vi "4.4 CSM API String to Numeric - TimeStamp.vi"() -> ()   [LabVIEW 2017]
uses:
  80786043-8302-4494-baed-a946b518dc40.vi
  b96edd05-43f6-4913-a4f3-d608f403e629.vi
  87278fde-cd95-4c12-a361-3a4a12f7c62e.vi
  36ad7d10-f589-4ebf-988f-4972958953c5.vi
  e1f6a09e-d061-4c8c-81e9-a26d802c807e.vi
  7cb491dc-0bc3-43bf-bfd1-0206b192279c.vi
  API-String-Arugments-Support/_Support/Convert API String Arguments to Data(variant).vi
  API-String-Arugments-Support/_Support/Data To API String Arguments.vi
  API-String-Arugments-Support/API String Arguments Support.lvlib
panel:
  out "output 4":T1={"Original"=timestamp(3779880873.3011937 s since 1904-01-01), "format string"="%<%Y-%m-%d %H:%M:%S>T", "CSM Timestamp Argument"="2023-10-11 22:54:33(%<%Y-%m-%d %H:%M:%S>T)", "Retrieved TimeStamp"=timestamp(3779880873 s since 1904-01-01), "Flatten String"="2023-10-11T14:54:33.000Z"}
  out "output 2":T2={"Argument String"="2023-10-31T14:49:39.597Z", "Type"=timestamp(0 s since 1904-01-01), "Retrieved TimeStamp"=timestamp(3781522179.597 s since 1904-01-01)}
  out "output 3":T3={"Original   "=timestamp(3781608579.597416 s since 1904-01-01), "Flatten String"="2023-10-31T14:49:39.597Z", "Type"=timestamp(0 s since 1904-01-01), "Retrieved TimeStamp"=timestamp(3781522179.597 s since 1904-01-01)}
  out "output 1":T2={"Argument String"="", "Type"=timestamp(0 s since 1904-01-01), "Retrieved TimeStamp"=timestamp(3839278850.481537 s since 1904-01-01)}
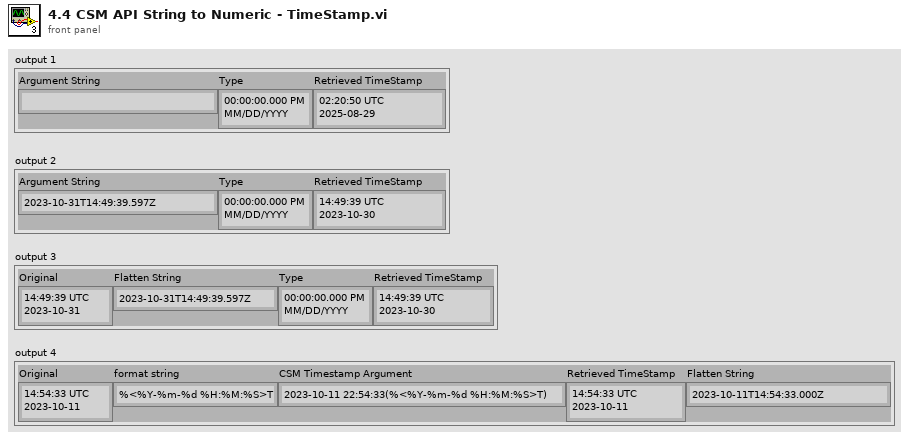
[diagram p1: front panel]
types:
  T1 = cluster{"Original":timestamp, "format string":string, "CSM Timestamp Argument":string, "Retrieved TimeStamp":timestamp, "Flatten String":string}
  T2 = cluster{"Argument String":string, "Type":timestamp, "Retrieved TimeStamp":timestamp}
  T3 = cluster{"Original   ":timestamp, "Flatten String":string, "Type":timestamp, "Retrieved TimeStamp":timestamp}
  T4 = cluster{"Empty String":string, "Type":timestamp, "Data":timestamp}
  T5 = cluster{"Arguments String":string, "Type":timestamp, "Data":timestamp}
  T6 = cluster{"Original   ":timestamp, "String":string, "Type":timestamp, "Data":timestamp}
  T7 = cluster{"Original":timestamp, "format string":string, "CSM Timestamp Argument":string, "Data":timestamp, "String":string}
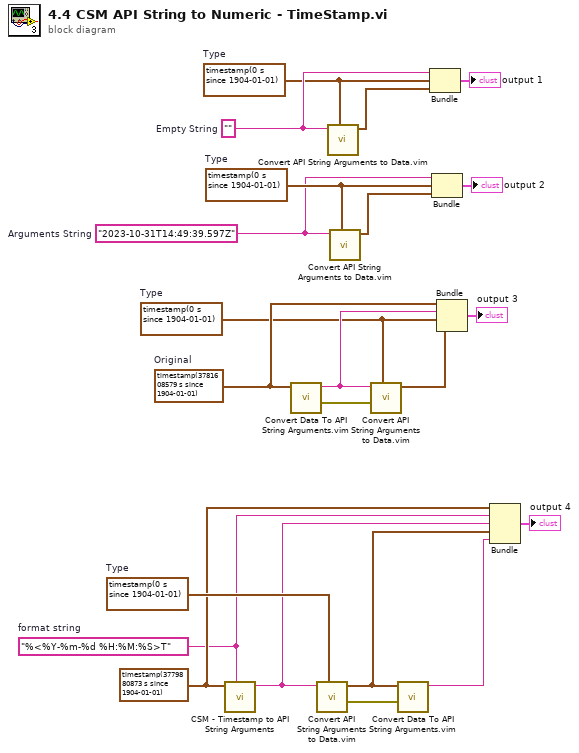
[diagram p0: block diagram]
diagram:
  w7 = timestamp(3779880873.3011937 s since 1904-01-01) ("Original")
  w9 = "2023-10-31T14:49:39.597Z"  # Arguments String
  w10 = timestamp(0 s since 1904-01-01)  # Type
  w15 = timestamp(0 s since 1904-01-01)  # Type
  w17 = timestamp(3781608579.597416 s since 1904-01-01)  # Original
  w22 = ""  # Empty String
  w21 = timestamp(0 s since 1904-01-01)  # Type
  w8 = timestamp(0 s since 1904-01-01)  # Type
  w6 = "%<%Y-%m-%d %H:%M:%S>T"  # format string
  n1 = call "CSM - Timestamp to API String Arguments.vi"("Format(Empty to use UTC)"=w6, "Timestamp (now)"=w7) -> ("CSM Timestamp Argument"=w5:string)  [unwired: 9 in]
  n2 = call "Convert Data To API String Arguments.vim"("data"=w17) -> ("error out"=w18:errorcluster, "String"=w16:string)  [unwired: 7 in]
  n3 = call "Convert API String Arguments to Data.vim"("Type"=w8, "String"=w5) -> ("error"=w4:errorcluster, "Data"=w3:timestamp)  [unwired: 6 in]
  n4 = call "Convert API String Arguments to Data.vim"("Type"=w21, "String"=w22) -> ("Data"=w20:timestamp)  [unwired: 6 in, 1 out]
  n5 = call "Convert API String Arguments to Data.vim"("Type"=w10, "String"=w9) -> ("Data"=w11:timestamp)  [unwired: 6 in, 1 out]
  n6 = call "Convert API String Arguments to Data.vim"("Type"=w15, "error in (no error)"=w18, "String"=w16) -> ("Data"=w14:timestamp)  [unwired: 5 in, 1 out]
  n7 = call "Convert Data To API String Arguments.vim"("error in (no error)"=w4, "data"=w3) -> ("String"=w2:string)  [unwired: 6 in, 1 out]
  n8 = Bundle("Empty String"=w22, "Type"=w21, "Data"=w20) -> (→"output 1":T4)  [unwired: 1 in]
  n9 = Bundle("Arguments String"=w9, "Type"=w10, "Data"=w11) -> (→"output 2":T5)  [unwired: 1 in]
  n10 = Bundle("Original"=w17, "String"=w16, "Type"=w15, "Data"=w14) -> (→"output 3":T6)  [unwired: 1 in]
  n11 = Bundle("Original"=w7, "format string"=w6, "CSM Timestamp Argument"=w5, "Data"=w3, "String"=w2) -> (→"output 4":T7)  [unwired: 1 in]
